vi "Log Data String.vi"(8 "error in (no error)":errorcluster, 10 "Log Data Cluster":T1, 11 "First Record":bool) -> (0 "error out":errorcluster, 3 "Log Data String":string)   [LabVIEW 2018, in "Logging.lvlib"]
uses:
  Logging.lvlib
  Log Data Cluster.ctl
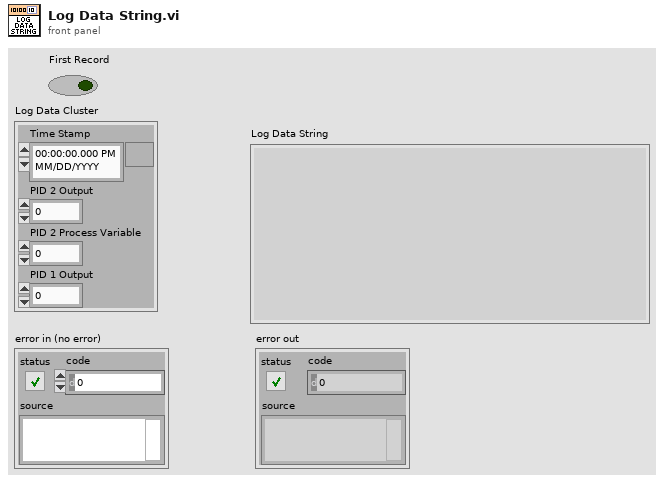
[diagram p1: front panel]
types:
  T1 = typedef "Logging.lvlib/Log Data Cluster.ctl" = cluster{"Time Stamp":timestamp, "PID 2 Output":dbl, "PID 2 Process Variable":dbl, "PID 1 Output":dbl}
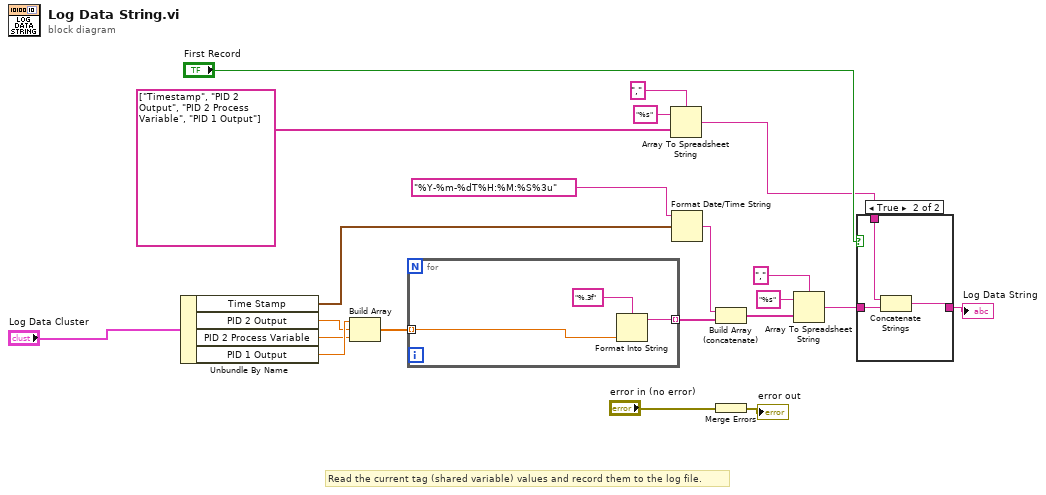
[diagram p0: block diagram]
diagram:
  # "Read the current tag (shared variable) values and record them to the log file."
  n1 = Unbundle By Name("Log Data Cluster") -> ("Time Stamp"=w6:timestamp, "PID 2 Output"=w16:dbl, "PID 2 Process Variable"=w15:dbl, "PID 1 Output"=w17:dbl)
  n2 = Build Array(w17, w16, w15) -> (w12:dbl[])
  n3 = for {
    tunnel: w12 -> [w22] mode=indexing
    tunnel: [w23] -> w8 mode=indexing
    n4 = Format Into String(format string="%.3f", w22) -> (resulting string=w23:string)  [unwired: 2 in, 1 out]
  }
  n5 = Array To Spreadsheet String(delimiter (Tab)=",", array=string[] ["Timestamp", "PID 2 Output", "PID 2 Process Variable", "PID 1 Output"] ("appended array"), 3:"%s" ("format string")) -> (spreadsheet string=w2:string)
  n6 = Format Date/Time String(time format string (%c)="%Y-%m-%dT%H:%M:%S%3u", seconds (now)=w6) -> (date/time string=w9:string)  [unwired: 1 in]
  n7 = Build Array (concatenate)(w9, w8) -> (w7:string[])
  n8 = Merge Errors("error in (no error)") -> (→"error out":errorcluster)
  n9 = Array To Spreadsheet String(delimiter (Tab)=",", array=w7, 3:"%s" ("format string")) -> (spreadsheet string=w13:string)
  n10 = case shown="True" "First Record" {
    tunnel: [w25 w28] -> w20
    tunnel: w13 -> [w25 w27]
    tunnel: w2 -> [_ w26]
    frame False {
    }
    frame True {
      n11 = Concatenate Strings(w26, w27) -> (w28:string)
    }
  }
  "Log Data String" <- w20
